vi "Untitled 5.vi"() -> ()   [LabVIEW 2021]
uses:
  <vilib>/Utility/miscctls.llb/LVBoundsTypeDef.ctl
panel:
  in  "a":i16
  in  "left corner":cluster{"horizontal":i16, "vertical":i16}
  out "new picture":picture
  in  "pixel center":cluster{"horizontal":i16, "vertical":i16}
  in  "radius":i16
  out "2D Picture":picture
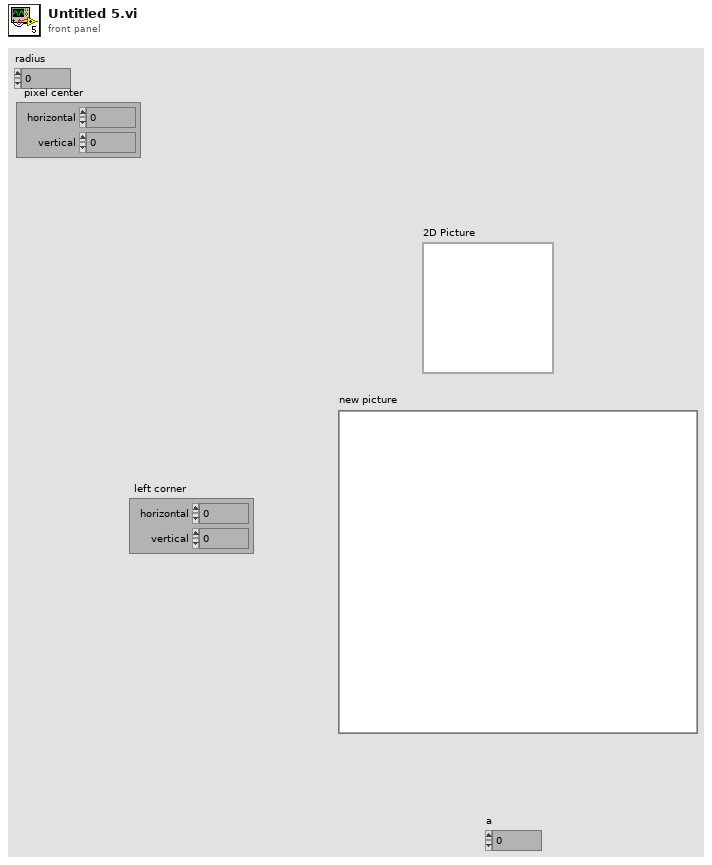
[diagram p1: front panel]
types:
  T1 = typedef "LVBoundsTypeDef.ctl" = cluster{"Width":u32, "Height":u32}
  T2 = cluster{"left":i16, "top":i16, "right":i16, "bottom":i16}
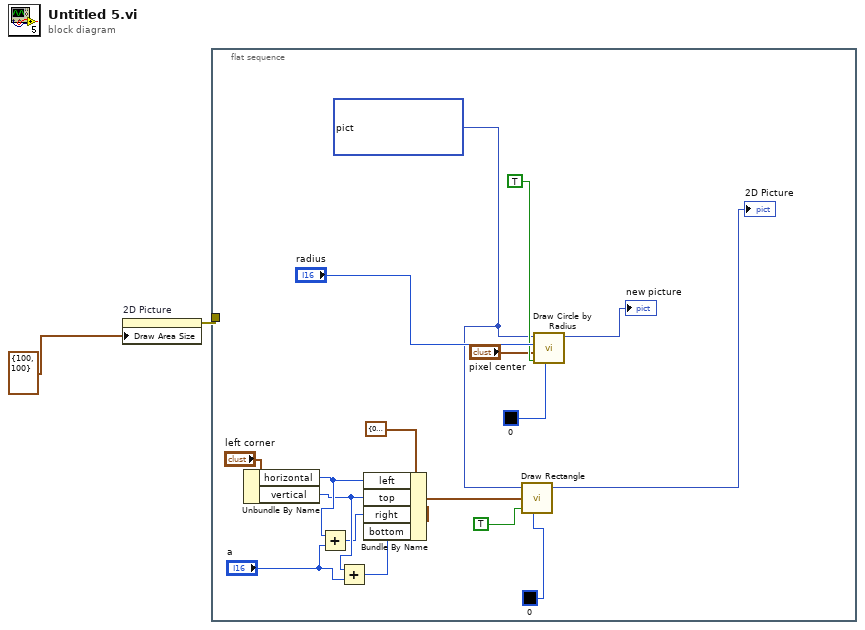
[diagram p0: block diagram]
diagram:
  n1 = property on="2D Picture" class="Pict"("Draw Area Size"=T1 {"Width"=100, "Height"=100}) -> (error out=w1:errorcluster)  [unwired: 2 in, 1 out]
  n2 = flat-sequence {
    tunnel: w1 -> [_]
    frame #0 {
      w13 = picture data[5B] ("picture")
      n3 = Unbundle By Name("left corner") -> ("horizontal"=w9:i16, "vertical"=w7:i16)
      n4 = Add(x=w9, y="a") -> (x+y=w6:i16)
      n5 = Add(x=w7, y="a") -> (x+y=w5:i16)
      n6 = Bundle By Name(cluster=T2 {"left"=0, "top"=0, "right"=0, "bottom"=0} ("rect"), "left"=w9, "top"=w7, "right"=w6, "bottom"=w5) -> (w10:T2)
      n7 = call <vilib>:"Draw Rectangle.vi"("picture"=w13, "rect"=w10, "fill?(F)"=TRUE, "color(black)"=u32 0) -> ("new picture"=→"2D Picture":picture)  [unwired: 5 in]
      n8 = call <vilib>:"Draw Circle by Radius.vi"("color(black)"=u32 0, "fill?(F)"=TRUE, "pixel center"="pixel center", "radius"="radius", "picture"=w13) -> ("new picture"=→"new picture":picture)  [unwired: 6 in]
    }
  }
